vi "kvCanGet4ByteChannelData.vi"(2 "error in (no error)":errorcluster, 3 "Data Item":T1(ring), 4 "Channel Number":i32) -> (0 "error out":errorcluster, 1 "Data":u32 format="%.0x")   [LabVIEW 2022 SP3]
doc: "This VI gets various 4-byte channel data values:\n\nItem \"Channel Capabilities\": the capabilities of the CAN controller; this is a combination of the canCHANNEL_CAP_xxx flags.\n\nItem \"Transceiver Capabilities\": the capabilities of the CAN transceiver; this is a combination of the canDRIVER_CAP_xxx flags.\n\nItem \"Channel Flags\": currently not implemented.\n\nItem \"Card Type\": the hardware type of the card. This value is any one of the canHWTYPE_xxx constants.\n\nItem \"Card Number\": the card's number in the computer. Each card type is numbered separately. For example, the first PCcan card in a machine will have number 0, the second PCcan number 1, etc. \n\nItem \"Channel Number On Card\": the channel number on the card."
uses:
  canlib32.dll
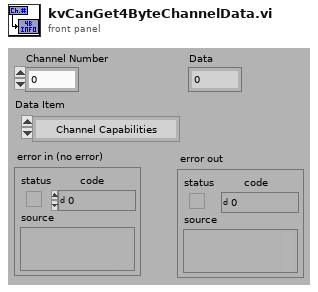
[diagram p1: front panel]
types:
  T1 = enum16{"Channel Capabilities", "Transceiver Capabilities", "Card Type", "Card Number", "Channel Number On Card"}
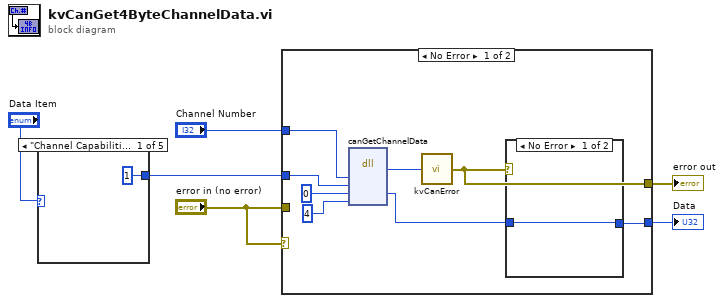
[diagram p0: block diagram]
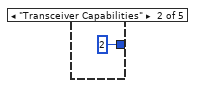
[diagram p2: hidden frame]
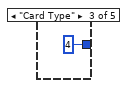
[diagram p3: hidden frame]
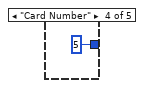
[diagram p4: hidden frame]
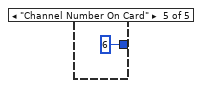
[diagram p5: hidden frame]
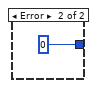
[diagram p6: hidden frame]
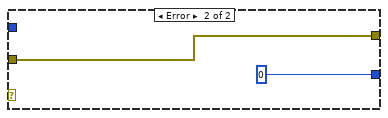
[diagram p7: hidden frame]
diagram:
  n1 = case shown="\"Channel Capabilities\", Default" "Data Item" {
    tunnel: [1 2 4 5 6] -> w1
    frame "Channel Capabilities", Default {
    }
    frame "Transceiver Capabilities" {
    }
    frame "Card Type" {
    }
    frame "Card Number" {
    }
    frame "Channel Number On Card" {
    }
  }
  n2 = case shown="No Error" "error in (no error)" {
    tunnel: "error in (no error)" -> [_ w23]
    tunnel: [w15 w23] -> w5
    tunnel: [w14 0] -> w4
    tunnel: "Channel Number" -> [w19 _]
    tunnel: w1 -> [w12 _]
    frame No Error {
      n3 = dll-call lib="canlib32.dll" fn="canGetChannelData" label="Call canGetChannelData"("channel"=w19, "item"=w12, "buffer"=0, "bufsize"=4) -> (w16:i32, "buffer"=w13:u32)  [unwired: 6 in, 2 out]
      n4 = call "kvCanError.vi"("error code"=w16) -> ("error out"=w15:errorcluster)
      n5 = case shown="No Error" w15 {
        tunnel: [w20 0] -> w14
        tunnel: w13 -> [w20 _]
        frame No Error {
        }
        frame Error {
        }
      }
    }
    frame Error {
    }
  }
  "error out" <- w5
  "Data" <- w4
